vi "Create Camera Index.vi"() -> (2 "Connection Ref":i32)   [LabVIEW 2024]
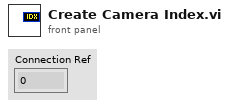
[diagram p1: front panel]
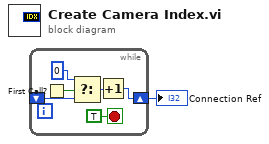
[diagram p0: block diagram]
diagram:
  n1 = while {
    shift-right: [w2] -> w1
    shift-left: _ -> [w5]
    stop <- TRUE stop-if-true
    n2 = First Call?() -> (First Call?: T/F=w6:bool)
    n3 = Select(t=0, s=w6, f=w5) -> (s? t:f=w3:i32)
    n4 = Increment(x=w3) -> (x+1=w2:i32)
  }
  "Connection Ref" <- w1
